vi "estadoToneBurst.vi"(8 "error in (no error)":errorcluster, 10 "Tm":i32=60, 11 "N":i32=1) -> (0 "error out":errorcluster)   [LabVIEW 2019, in "Prueba31.lvclass"]
uses:
  Prueba31.lvclass
panel:
  out "Tm":i32=60
  out "seg":i32=60
  in  "terminar":bool
  out "N_actual":i32
  out "N":i32=1
  out "estado":string
  # "Repeticiones que debe hacer"
  # "Repetición actual"
  # "Tiempo de la prueba"
  # "Segundos"
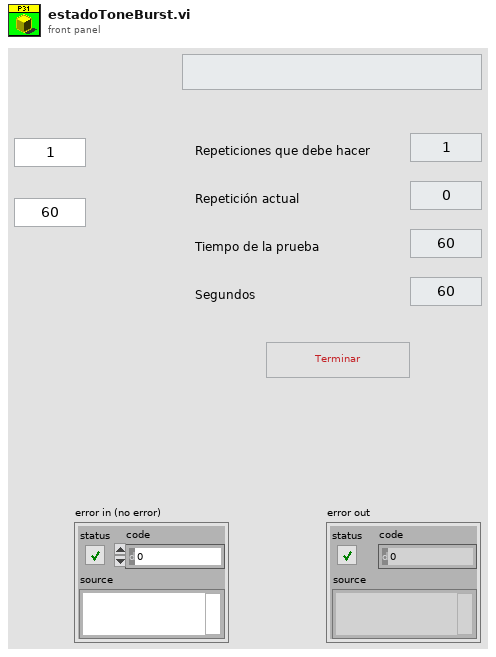
[diagram p1: front panel]
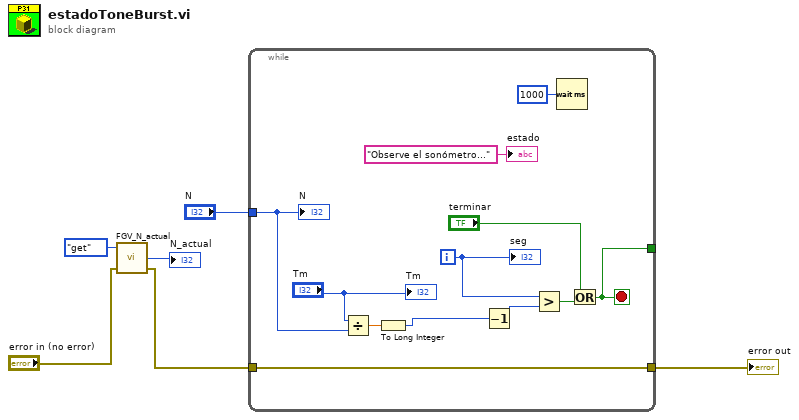
[diagram p0: block diagram]
diagram:
  n1 = call "FGV_N_actual.vi"("error in (no error)"="error in (no error)", "action"=enum16{"increment", "set_start", "get"}."get") -> ("error out"=w2:errorcluster, "N_actual out"=→"N_actual":i32)  [unwired: 2 in]
  n2 = while {
    tunnel: [w13] -> _
    tunnel: "N" -> [w9]
    tunnel: w2 -> [w11]
    tunnel: [w11] -> w1
    i -> [w17]
    stop <- w13 stop-if-true
    n3 = Divide(x="Tm", y=w9) -> (x/y=w8:dbl)
    n4 = To Long Integer(number=w8) -> (32bit integer=w7:i32)
    n5 = Decrement(x=w7) -> (x-1=w12:i32)
    n6 = Greater?(x=w17, y=w12) -> (0:w15:bool)
    n7 = Wait (ms)(milliseconds to wait=u32 1000) -> ()  [unwired: 1 out]
    n8 = Or(x="terminar", y=w15) -> (x .or. y?=w13:bool)
    "estado" <- "Observe el sonómetro..." ("estado")
    "seg" <- w17
    "N" <- w9
    "Tm" <- "Tm"
  }
  "error out" <- w1
